vi "Digest Error.vi"(8 "error in (no error)":errorcluster, 10 "TALOS Error In":T1 {"Time Stamp" format="%<%x %.3X>T"}, 11 "Error Manager in":refnum<class "Error Manager.lvclass">) -> (0 "error out":errorcluster, 3 "Error Manager out":refnum<class "Error Manager.lvclass">)   [LabVIEW 2026, in "TALOS.lvlib" / "Error Manager.lvlib" / "Error Manager.lvclass"]
uses:
  Error Manager.lvclass
  C:/LabVIEW Code/TALOS/talos/Father of all uServices/Father of all uServices/Father of all uServices.lvclass
  Error Info.ctl
  <vilib>/Utility/error.llb/DialogType.ctl
  Guardian/Guardian Messages/Message to uService Msg/Message to uService Msg.lvclass/Message to uService Msg.ctl
  Ancestor/Ancestor/Ancestor.lvclass/Ancestor.ctl
  FGV/Error Memory/Get All Errors Arrays.vi
  FGV/Error Memory/Error Memory Core.vi
  Guardian/Guardian Messages/Message to uService Msg/Send Message to uService.vi
  Support VIs/Generate Error.vi
  Support VIs/Circus Root Path.vi
  FGV/Error Memory/Error Crt Lvl checker.vi
  FGV/Error Memory/Error Memory Core.vi/40c8088d-b597-4017-91af-faa98e00292e.vi
  FGV/Error Memory/Error Memory Core.vi/d4a3ab98-063c-4e44-b43d-fbdcfe6c2be2.vi
  FGV/Error Memory/Get Error Description.vi
  Support VIs/Get PC name.vi
  Ancestor/Ancestor/Read ID.vi
  Support VIs/Get Class Name.vi
  <vilib>/Utility/error.llb/Clear Errors.vi
  <vilib>/AdvancedString/Delimited String to 1D String Array.vi
  <vilib>/AdvancedString/Delimited String to 1D String Array (string).vi
  Father of all uServices/Father of all uServices/Father of all uServices.lvclass
  C:/LabVIEW Code/TALOS/builds/Actor Framework PPL/Actor Framework.lvlibp/1abvi3w/vi.lib/ActorFramework/Actor/Actor.lvclass
  Support VIs/TALOS Root path.vi
  Support VIs/Read CSV worksheet.vi
  Support VIs/Global Memory.vi
  Support VIs/Global Constants.vi
  <vilib>/Utility/error.llb/General Error Handler.vi
  builds/Actor Framework PPL/Actor Framework.lvlibp/1abvi3w/vi.lib/ActorFramework/Actor/Read Caller Enqueuer.vi
  builds/Actor Framework PPL/Actor Framework.lvlibp/1abvi3w/vi.lib/ActorFramework/Message Enqueuer/Enqueue.vi
  <vilib>/Utility/LVClass/Get LV Class Name.vi
  Support VIs/Error Log.vi
  <vilib>/Comparison/Equal/Equal Functor/Equal Functor.lvclass
  Guardian/Guardian Messages/Message to uService Msg/Message to uService Msg.lvclass
  Ancestor/Ancestor/Ancestor.lvclass
  Classes/Error Filter/Error Filter.lvclass
  TALOS.lvlib
  FGV/Error Memory/Error Memory.lvlib
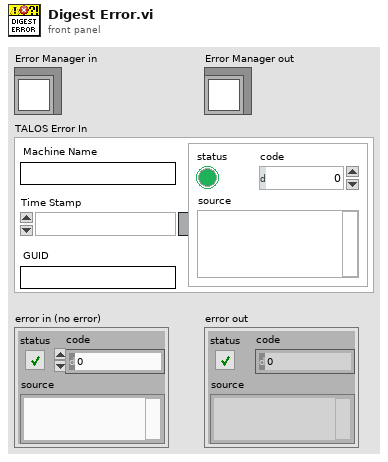
[diagram p1: front panel]
types:
  T1 = typedef "TALOS.lvlib/Error Manager.lvlib/Error Manager.lvclass/Error Info.ctl" = cluster{"error out":errorcluster, "Time Stamp":timestamp, "Machine Name":string, "GUID":string}
  T2 = typedef "DialogType.ctl" = u16
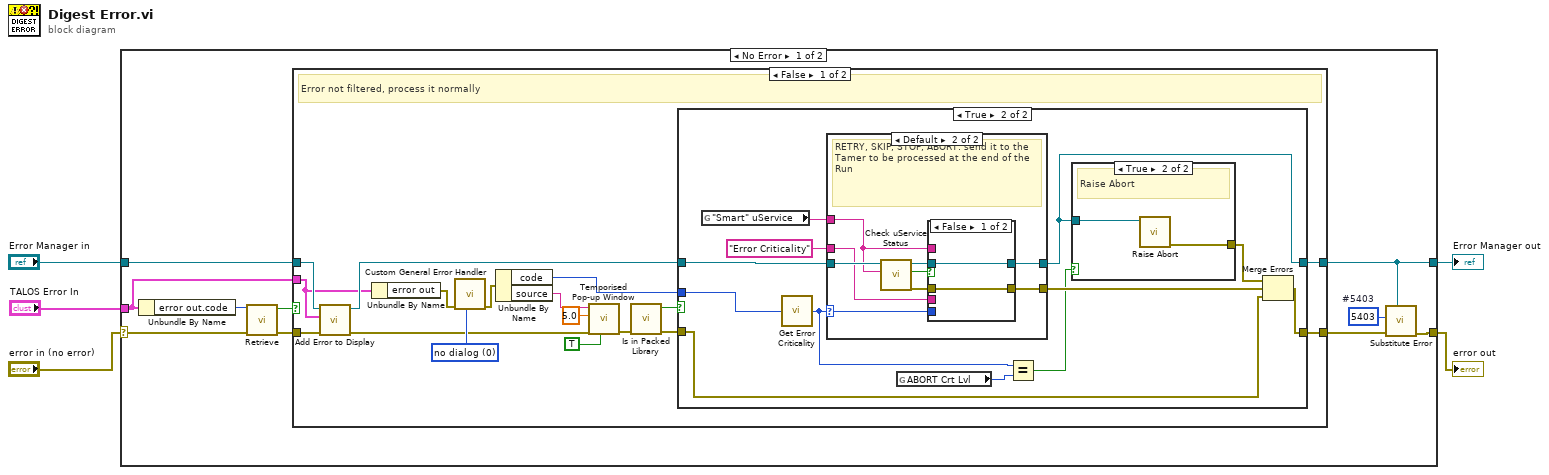
[diagram p0: block diagram]
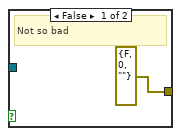
[diagram p3: hidden frame]
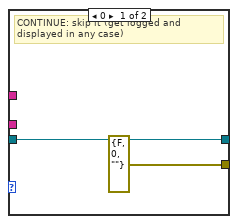
[diagram p4: hidden frame]
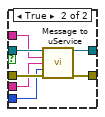
[diagram p5: hidden frame]
diagram:
  n1 = case shown="No Error" "error in (no error)" {
    selector: "error in (no error)" -> [w11 w72]
    tunnel: "TALOS Error In" -> [w10 _]
    tunnel: "Error Manager in" -> [w13 w73]
    tunnel: [w7 w72] -> w1
    tunnel: [w6 w73] -> w5
    frame No Error {
      w9 = 5403  # #5403
      n2 = Unbundle By Name(w10) -> ("error out.code"=w12:i32)
      n3 = call "Retrieve.vi"("error in (no error)"=w11, "Error Code"=w12) -> ("error out"=w15:errorcluster, "Filter?"=w14:bool)  [unwired: 8 in]
      n4 = case shown="False" w14 {
        tunnel: w13 -> [w27 w71]
        tunnel: [w32 w71] -> w6
        tunnel: [w31 w70] -> w8
        tunnel: w15 -> [w29 w70]
        tunnel: w10 -> [w24 _]
        frame False {
          w26 = T2 0 items=["no dialog", "OK message", "continue or stop message", "OK message + warnings", "continue/stop + warnings"] ("type of dialog (OK msg:1)")
          # "Error not filtered, process it normally"
          n5 = call "Add Error to Display.vi"("error in (no error)"=w29, "error to display"=w24, "Error Manager in"=w27) -> ("error out"=w25:errorcluster, "Error Manager out"=w28:refnum<class "Error Manager.lvclass">)  [unwired: 7 in]
          n6 = Unbundle By Name(w24) -> ("error out"=w23:errorcluster)
          n7 = call "Custom General Error Handler.vi"("type of dialog (OK msg:1)"=w26, "error in (no error)"=w23) -> ("error out"=w20:errorcluster)  [unwired: 9 in]
          n8 = Unbundle By Name(w20) -> ("code"=w22:i32, "source"=w21:string)
          n9 = call "Temporised Pop-up Window.vi"("error window"=TRUE, "error in (no error)"=w25, "Timeout"=5.0, "Text"=w21) -> ("error out"=w19:errorcluster)  [unwired: 7 in]
          n10 = call "Is in Packed Library.vi"("error in (no error)"=w19) -> ("error out"=w17:errorcluster, "Is In Packed Library"=w18:bool)  [unwired: 9 in]
          n11 = case shown="True" w18 {
            tunnel: [w34 w35] -> w32
            tunnel: [w33 w46] -> w31
            tunnel: w28 -> [w34 w42]
            tunnel: w22 -> [_ w41]
            tunnel: w17 -> [w33 w40]
            frame False {
            }
            frame True {
              n12 = global read "Global Constants.vi" "\"Smart\" uService"() -> (w43:string)
              n13 = call "Get Error Criticality.vi"("Error Code in"=w41) -> ("Error Criticality"=w38:u8)  [unwired: 4 in]
              n14 = case shown="Default" w38 {
                selector: w38 -> [_ w54]
                tunnel: w42 -> [w51 w56]
                tunnel: [w51 w59] -> w35
                tunnel: [errorcluster {"status"=FALSE, "code"=0, "source"=""} ("error out") w60] -> w45
                tunnel: "Error Criticality" ("Message") -> [_ w55]
                tunnel: w43 -> [_ w53]
                frame 0 {
                  # "CONTINUE: skip it (get logged and displayed in any case)"
                }
                frame Default {
                  # "RETRY, SKIP, STOP, ABORT: send it to the Tamer to be processed at the end of the Run"
                  n15 = call-dynamic "Check uService Status.vi"("uService ID"=w53, "Father of all uServices in"=w56) -> ("error out"=w57:errorcluster, "Online?"=w52:bool, "Father of all uServices out"=w58:refnum<class "Error Manager.lvclass">)  [unwired: 6 in, 1 out]
                  n16 = case shown="False" w52 {
                    tunnel: [w61 w69] -> w60
                    tunnel: [w62 w68] -> w59
                    tunnel: w58 -> [w62 w67]
                    tunnel: w57 -> [w61 w66]
                    tunnel: w55 -> [_ w65]
                    tunnel: w54 -> [_ w64]
                    tunnel: w53 -> [_ w63]
                    frame False {
                    }
                    frame True {
                      n17 = call "Message to uService.vi"("Father of all uServices in"=w67, "uService ID"=w63, "Message"=w65, "Data"=w64, "error in (no error)"=w66) -> ("Father of all uServices out"=w68:refnum<class "Error Manager.lvclass">, "error out"=w69:errorcluster)  [unwired: 9 in]
                    }
                  }
                }
              }
              n18 = global read "Global Constants.vi" "ABORT Crt Lvl"() -> (w39:u8)
              n19 = Equal?(x=w38, y=w39) -> (x = y?=w37:bool)
              n20 = case shown="True" w37 {
                tunnel: [errorcluster {"status"=FALSE, "code"=0, "source"=""} ("error out") w48] -> w36
                tunnel: w35 -> [_ w49]
                frame False {
                  # "Not so bad"
                }
                frame True {
                  # "Raise Abort"
                  n21 = call "Raise Abort.vi"("Father of all uServices in"=w49) -> ("error out"=w48:errorcluster)  [unwired: 9 in, 1 out]
                }
              }
              n22 = Merge Errors(w36, w45, w40) -> (w46:errorcluster)
            }
          }
        }
        frame True {
          # "Error filtered, skip it"
        }
      }
      n23 = call "Substitute Error.vi"("LabVIEW Object"=w6, "error in (no error)"=w8, "Error Code"=w9) -> ("error out"=w7:errorcluster)  [unwired: 8 in]
    }
    frame Error {
    }
  }
  "Error Manager out" <- w5
  "error out" <- w1
